vi "KE6221 -- Get Wave External Trig Params.vi"(0 "Resource In":refnum<visa-resource-name>, 1 "Check For SCPI Errors? (T)":bool=TRUE, 11 "error in (no error)":errorcluster) -> (4 "Resource Out (dupl)":refnum<visa-resource-name>, 8 "External Trig Params":T1={"Ext Trig Enabled?"=FALSE, "Trig Link In Line"=enum."None", "Inactive Level (%)"=50.0, "Ignore Retrigs?"=FALSE} {"Inactive Level (%)" min=-100.0 max=100.0 format="%.3p"}, 15 "error out":errorcluster)   [LabVIEW 2019, in "Keithley 622x.lvlib"]
doc: "Returns the trigger parameters for waveform playback. Note that this VI can only be used with the 6221, since the 6220 doesn't support this feature."
uses:
  Keithley 622x.lvlib
  Typedefs/KE6221 -- Wave External Trig Params.ctl
  Low Level/Typedefs/KE6221 -- Wave Extern Trig Link In Line.ctl
  Low Level/Typedefs/KE6221 -- Wave Inactive Level.ctl
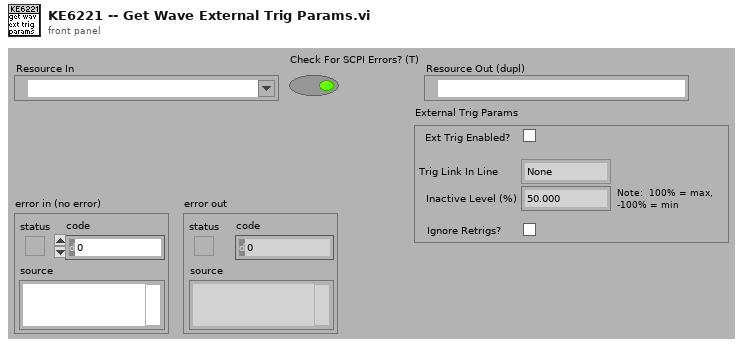
[diagram p1: front panel]
types:
  T1 = typedef "Keithley 622x.lvlib/KE6221 -- Wave External Trig Params.ctl" = cluster{"Ext Trig Enabled?":bool, "Trig Link In Line":T2, "Inactive Level (%)":T3, "Ignore Retrigs?":bool}
  T2 = typedef "Keithley 622x.lvlib/KE6221 -- Wave Extern Trig Link In Line.ctl" = enum16{"None", "1", "2", "3", "4", "5", "6"}
  T3 = typedef "Keithley 622x.lvlib/KE6221 -- Wave Inactive Level.ctl" = dbl
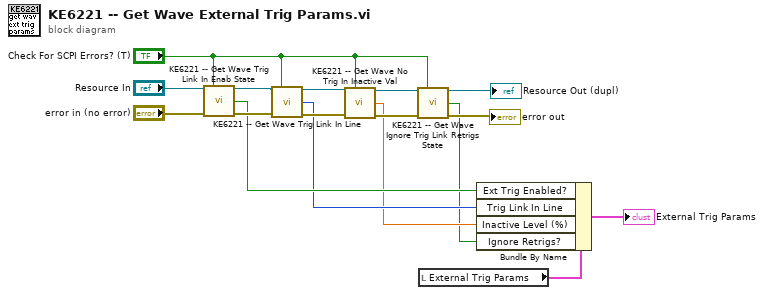
[diagram p0: block diagram]
diagram:
  n1 = call "KE6221 -- Get Wave Trig Link In Enab State.vi"("Resource In"="Resource In", "Check For SCPI Errors? (T)"="Check For SCPI Errors? (T)", "error in (no error)"="error in (no error)") -> ("Resource Out (dupl)"=w15:refnum<visa-resource-name>, "Trig Link In Enabled?"=w5:bool, "error out"=w14:errorcluster)  [unwired: 10 in]
  n2 = call "KE6221 -- Get Wave Trig Link In Line.vi"("Resource In"=w15, "Check For SCPI Errors? (T)"="Check For SCPI Errors? (T)", "error in (no error)"=w14) -> ("Resource Out (dupl)"=w13:refnum<visa-resource-name>, "Trig Link In Line"=w4:T2, "error out"=w12:errorcluster)  [unwired: 10 in]
  n3 = call "KE6221 -- Get Wave No Trig In Inactive Val.vi"("Resource In"=w13, "Check For SCPI Errors? (T)"="Check For SCPI Errors? (T)", "error in (no error)"=w12) -> ("Resource Out (dupl)"=w11:refnum<visa-resource-name>, "Inactive Level (%)"=w3:T3, "error out"=w10:errorcluster)  [unwired: 10 in]
  n4 = call "KE6221 -- Get Wave Ignore Trig Link Retrigs State.vi"("Resource In"=w11, "Check For SCPI Errors? (T)"="Check For SCPI Errors? (T)", "error in (no error)"=w10) -> ("Resource Out (dupl)"=→"Resource Out (dupl)":refnum<visa-resource-name>, "Ignore Retrigs?"=w2:bool, "error out"=→"error out":errorcluster)  [unwired: 10 in]
  n5 = local read "External Trig Params"() -> (w6:T1)
  n6 = Bundle By Name(cluster=w6, "Ext Trig Enabled?"=w5, "Trig Link In Line"=w4, "Inactive Level (%)"=w3, "Ignore Retrigs?"=w2) -> (→"External Trig Params":T1)
